vi "ARCO Read Client.vi"() -> ()   [LabVIEW 2017]
uses:
  <vilib>/OPCUA/controls/NodeIds.ctl
  <vilib>/OPCUA/controls/NodeId.ctl
  <vilib>/OPCUA/NI OPC UA Client.lvlib
panel:
  in  "stop":bool
  out "error out":errorcluster
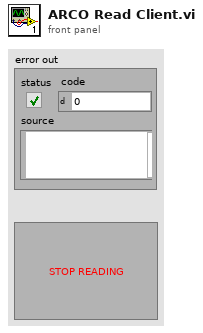
[diagram p1: front panel]
types:
  T1 = cluster{"message mode":enum16{"None", "Sign", "Sign and Encrypt"}, "security":enum16{"Basic256", "Basic128Rsa15"}}
  T2 = typedef "NodeIds.ctl" = T3[]
  T3 = typedef "NodeId.ctl" = string
  T4 = typedef "OPC UA Client Refnum.ctl" = refnum<k21>
  T5 = typedef "Subscription ID.ctl" = u32
  T6 = typedef "Subscription Data Change.ctl" = cluster{"node ID":T3, " value":variant, "timestamp":timestamp, "data type":T7, "status code":T8}
  T7 = typedef "Data Type.ctl" = u16
  T8 = typedef "OPC UA StatusCode.ctl" = u32
  T9 = cluster{"[0]":sgl, "[1]":sgl, "[2]":sgl, "[3]":sgl, "[4]":sgl, "[5]":sgl, "[6]":sgl, "[7]":sgl, "[8]":sgl, "[9]":sgl, "[10]":sgl, "[11]":sgl, "[12]":sgl, "[13]":sgl, "[14]":sgl, "[15]":sgl, "[16]":sgl, "[17]":sgl, "[18]":sgl, "[19]":sgl, "[20]":sgl, "[21]":sgl, "[22]":sgl, "[23]":sgl, "[24]":sgl, "[25]":sgl, "[26]":sgl, "[27]":sgl, "[28]":sgl, "[29]":sgl, "[30]":sgl, "[31]":sgl, "[32]":sgl, "[33]":sgl, "[34]":sgl, "[35]":sgl, "[36]":sgl, "[37]":sgl, "[38]":sgl, "[39]":sgl, "[40]":sgl, "[41]":sgl, "[42]":sgl, "[43]":sgl, "[44]":sgl, "[45]":sgl, "[46]":sgl, "[47]":sgl, "[48]":sgl, "[49]":sgl, "[50]":sgl, "[51]":sgl, "[52]":sgl, "[53]":sgl, "[54]":sgl, "[55]":sgl, "[56]":sgl, "[57]":sgl, "[58]":sgl, "[59]":sgl, "[60]":sgl, "[61]":sgl, "[62]":sgl}
  T10 = cluster{"[0]":bool, "[1]":bool, "[2]":bool, "[3]":bool, "[4]":bool, "[5]":bool, "[6]":bool, "[7]":bool, "[8]":bool, "[9]":bool, "[10]":bool, "[11]":bool, "[12]":bool, "[13]":bool, "[14]":bool, "[15]":bool, "[16]":bool, "[17]":bool, "[18]":bool, "[19]":bool, "[20]":bool, "[21]":bool, "[22]":bool, "[23]":bool, "[24]":bool, "[25]":bool, "[26]":bool, "[27]":bool, "[28]":bool, "[29]":bool, "[30]":bool, "[31]":bool, "[32]":bool, "[33]":bool, "[34]":bool, "[35]":bool, "[36]":bool, "[37]":bool, "[38]":bool, "[39]":bool, "[40]":bool, "[41]":bool, "[42]":bool, "[43]":bool, "[44]":bool, "[45]":bool, "[46]":bool, "[47]":bool, "[48]":bool, "[49]":bool, "[50]":bool, "[51]":bool, "[52]":bool, "[53]":bool, "[54]":bool, "[55]":bool, "[56]":bool, "[57]":bool, "[58]":bool, "[59]":bool, "[60]":bool, "[61]":bool, "[62]":bool}
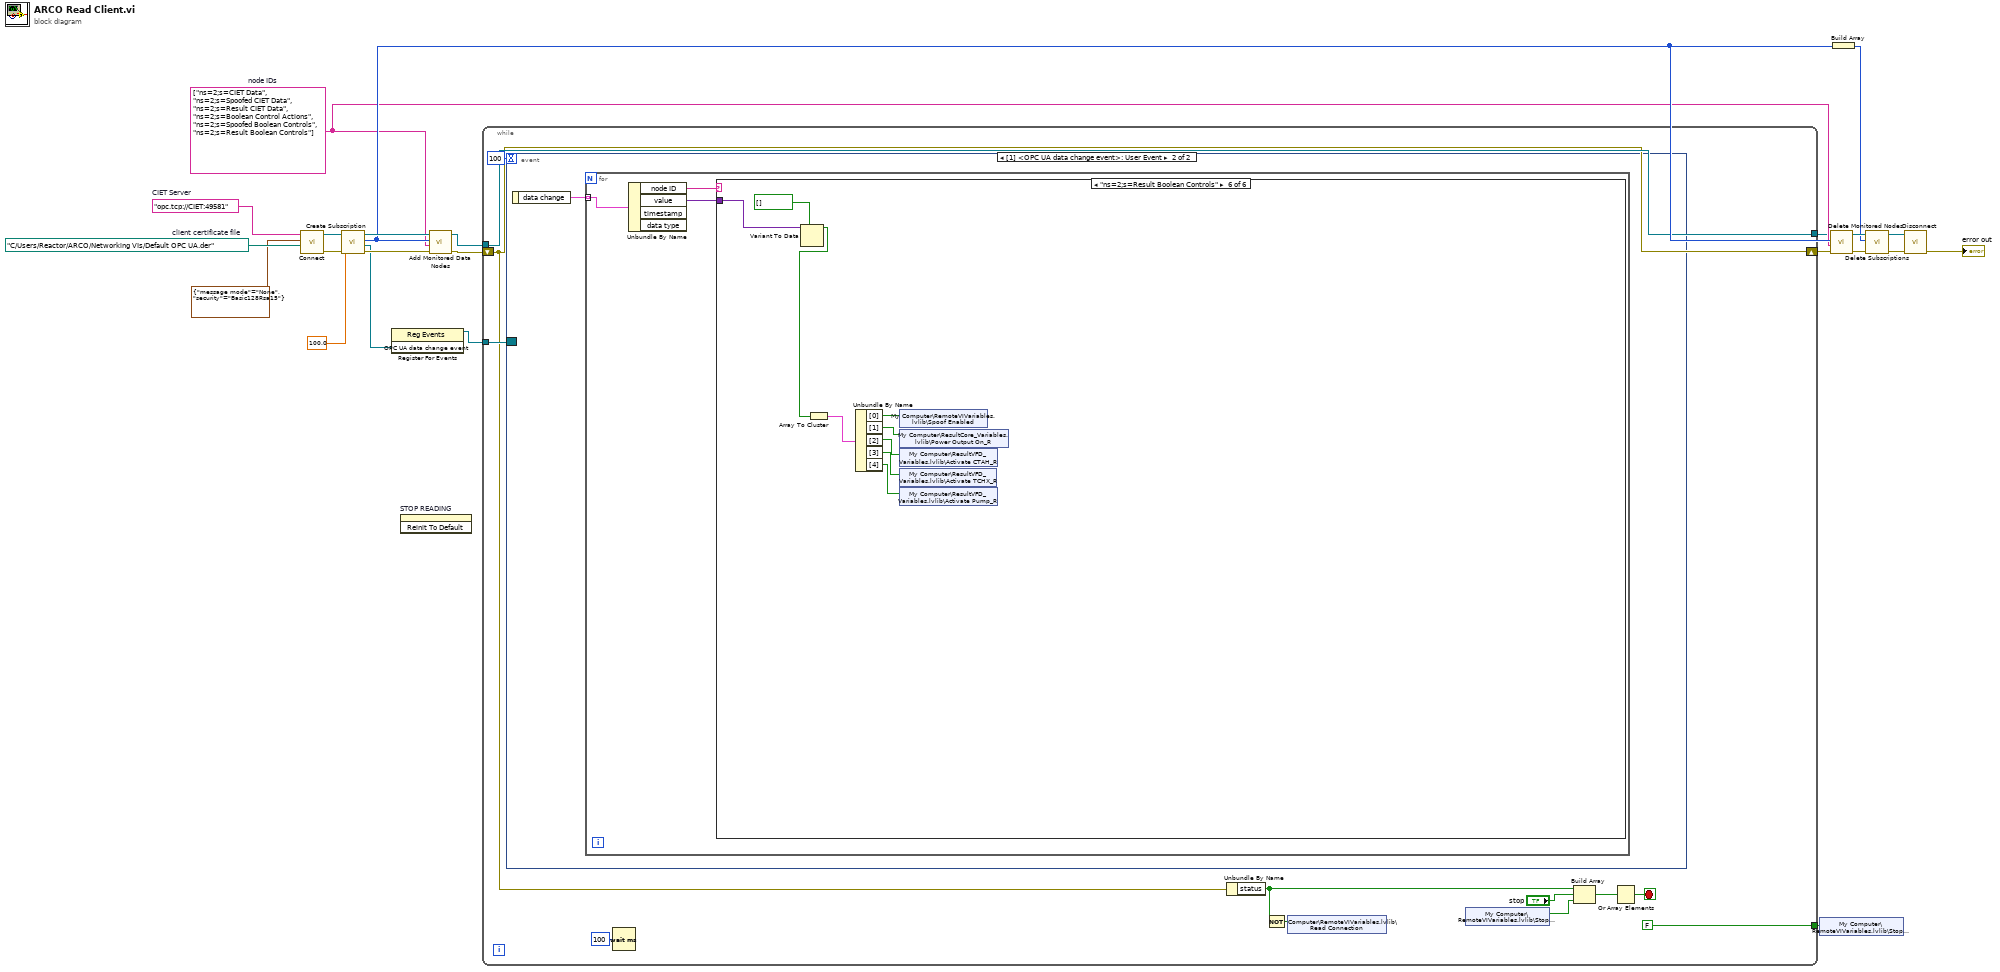
[diagram p0: block diagram]
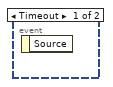
[diagram p2: hidden frame]
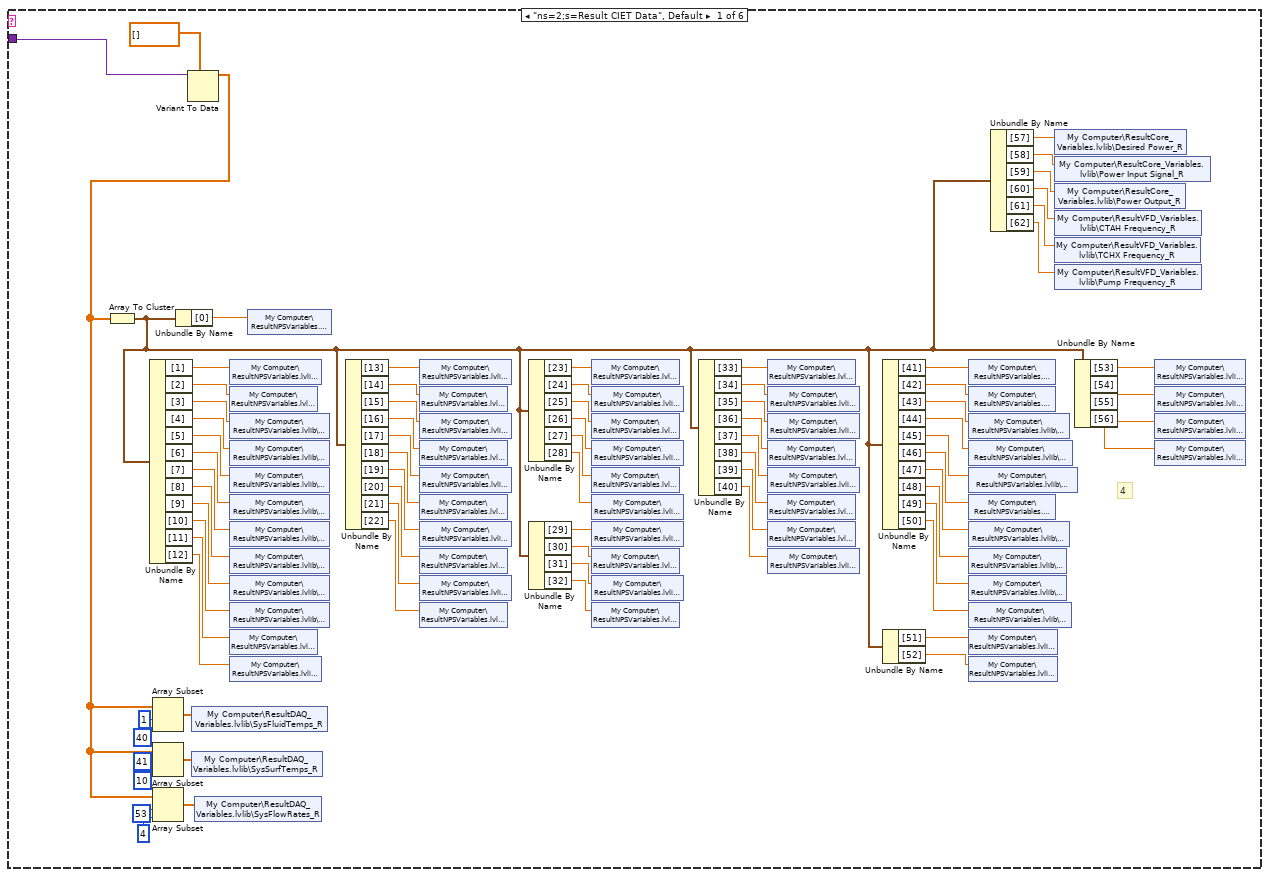
[diagram p3: hidden frame]
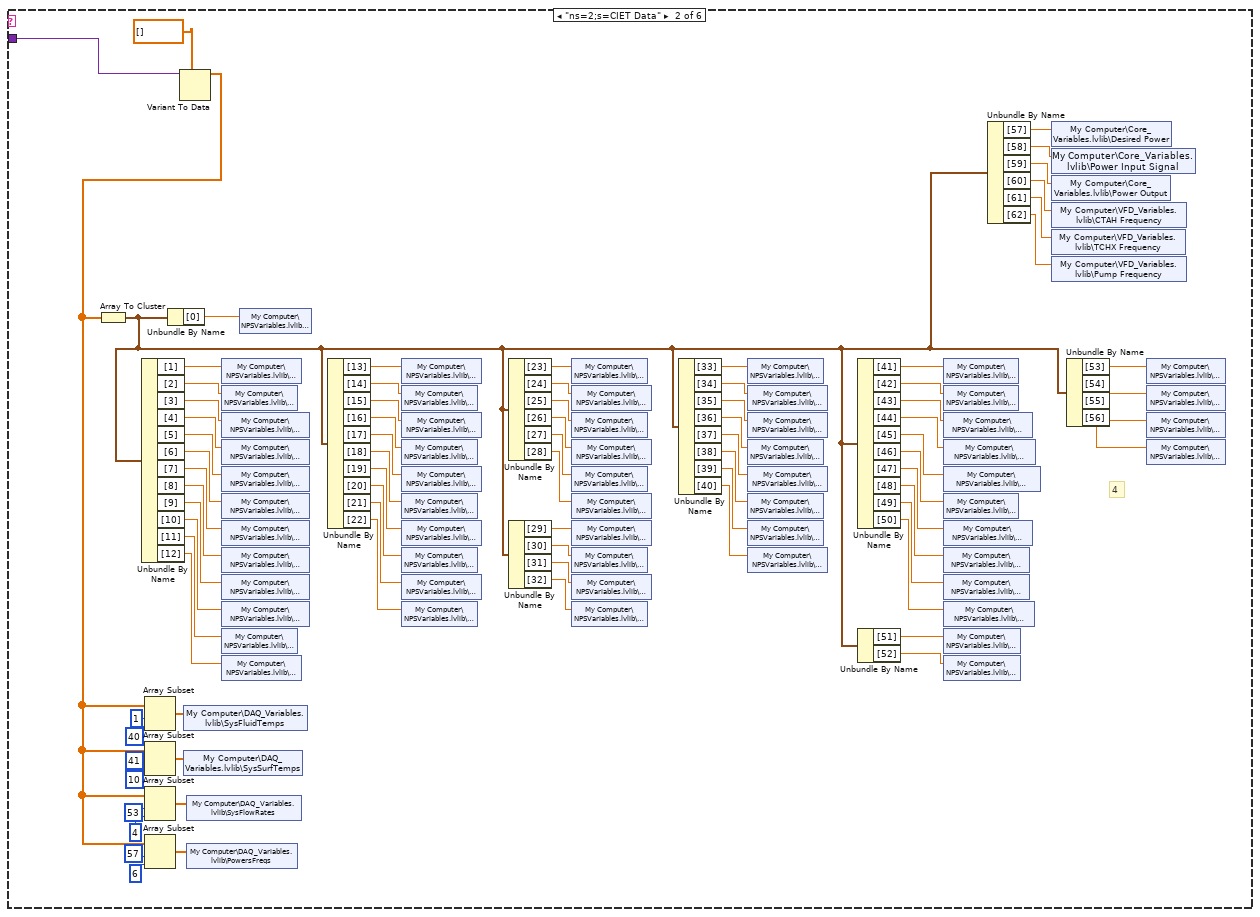
[diagram p4: hidden frame]
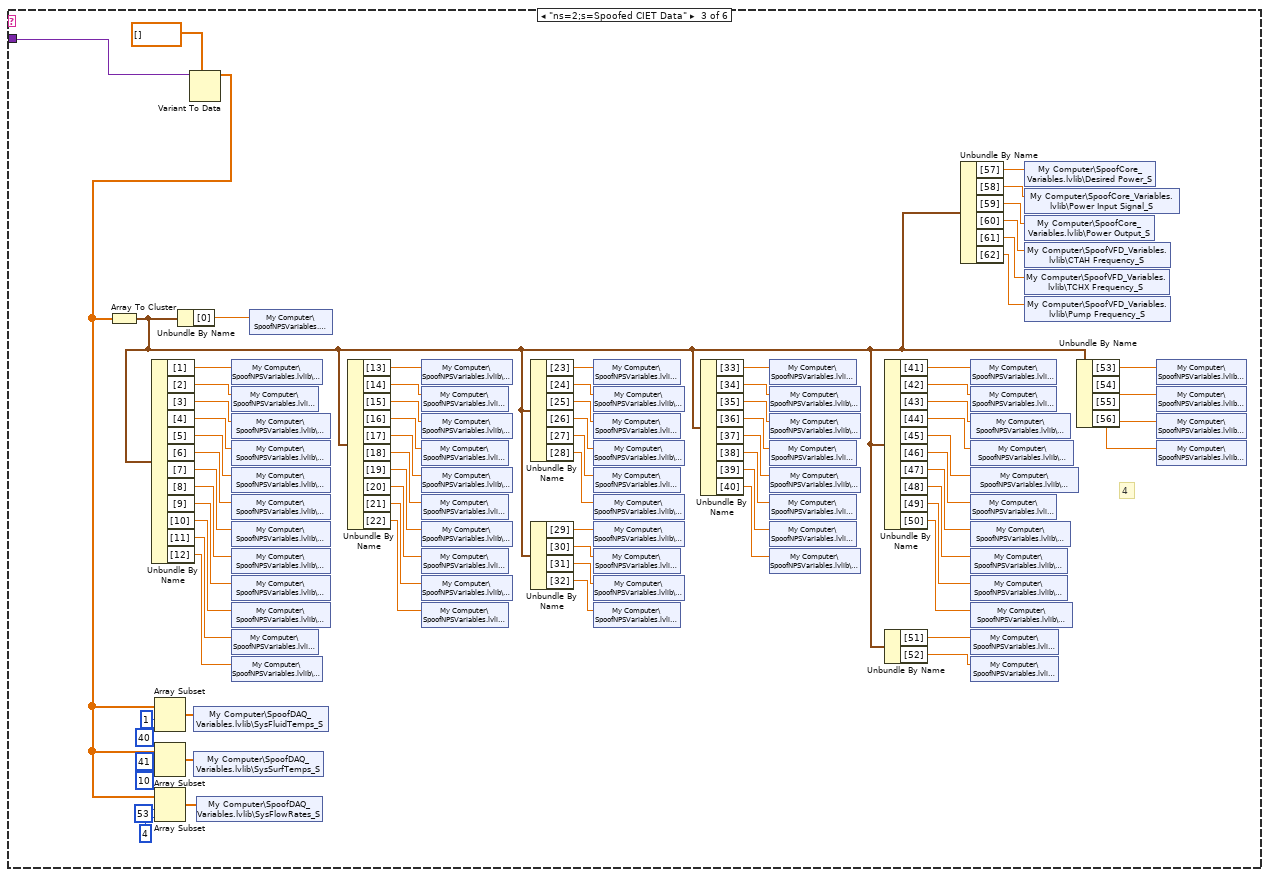
[diagram p5: hidden frame]
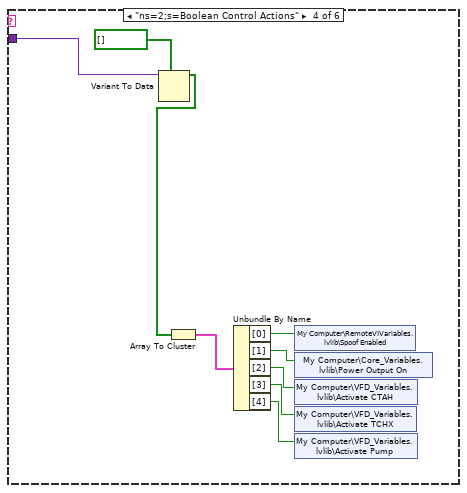
[diagram p6: hidden frame]
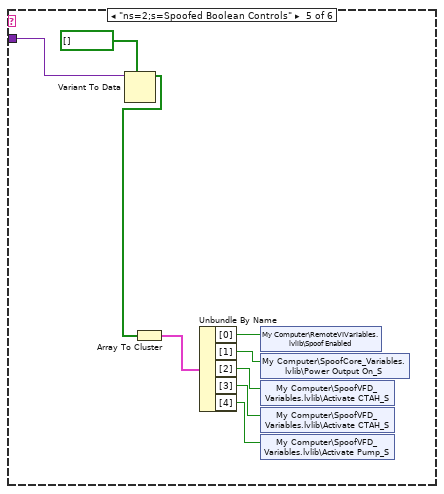
[diagram p7: hidden frame]
diagram:
  w7 = T2 ["ns=2;s=CIET Data", "ns=2;s=Spoofed CIET Data", "ns=2;s=Result CIET Data", "ns=2;s=Boolean Control Actions", "ns=2;s=Spoofed Boolean Controls", "ns=2;s=Result Boolean Controls"]  # node IDs
  w21 = path "C:/Users/Reactor/ARCO/Networking VIs/Default OPC UA.der"  # client certificate file
  w22 = "opc.tcp://CIET:49581"  # CIET Server
  n1 = call <vilib>:"Connect.vi"("client certificate file"=w21, "security policy"=T1 {"message mode"=enum."None", "security"=enum."Basic128Rsa15"}, "server endpoint URL"=w22) -> ("error out"=w3:errorcluster, "OPC UA client refnum out"=w19:T4)  [unwired: 6 in, 1 out]
  n2 = call <vilib>:"Create Subscription.vi"("error in (no error)"=w3, "publishing interval (1000 ms)"=100.0, "OPC UA client refnum in"=w19) -> ("error out"=w17:errorcluster, "OPC UA data change event"=w16:refnum<user-event>, "subscription ID out"=w11:T5, "OPC UA client refnum out"=w18:T4)  [unwired: 4 in, 1 out]
  n3 = register-events(w16) -> (reference out=w9:refnum<event-registration>)  [unwired: 2 in, 1 out]
  n4 = invoke on="STOP READING" class="Bool (strict)" method="Reinit To Default"() -> ()  [unwired: 3 in, 3 out]
  n5 = call <vilib>:"Add Monitored Data Nodes.vi"("error in (no error)"=w17, "node IDs"=w7, "subscription ID in"=w11, "OPC UA client refnum in"=w18) -> ("error out"=w2:errorcluster, "OPC UA client refnum out"=w8:T4)  [unwired: 4 in, 2 out]
  n6 = while {
    tunnel: w9 -> [w35]
    tunnel: w8 -> [w33]
    tunnel: [w33] -> w6
    tunnel: [FALSE] -> w4
    shift-right: [w24] -> w1
    shift-left: w2 -> [w24]
    stop <- w25 stop-if-true
    n7 = event shown="[1] <OPC UA data change event>: User Event" {
      selector: w35 -> [_ _]
      dyn-events: _ -> [_ _]
      timeout: 100 -> [_ _]
      event Timeout {
        n8 = event-data() -> ()  [unwired: 1 in, 1 out]
      }
      event User Event {
        n9 = event-data() -> ("data change"=w36:T6[])  [unwired: 1 in]
        n10 = for {
          tunnel: w36 -> [w38] mode=indexing
          n11 = Unbundle By Name(w38) -> ("node ID"=w37:T3, "value"=w39:variant)  [unwired: 2 out]
          n12 = case shown="\"ns=2;s=Result Boolean Controls\"" w37 {
            tunnel: w39 -> [w49 w135 w203 w271 w280 w289]
            frame "ns=2;s=Result CIET Data", Default {
              # "4"
              n13 = Variant To Data(type=sgl[] [], Variant=w49) -> (data=w47:sgl[])  [unwired: 1 in, 1 out]
              n14 = Array To Cluster(array=w47) -> (cluster=w40:T9)
              n15 = Unbundle By Name(w40) -> ("[1]"=w56:sgl, "[2]"=w58:sgl, "[3]"=w59:sgl, "[4]"=w60:sgl, "[5]"=w61:sgl, "[6]"=w62:sgl, "[7]"=w63:sgl, "[8]"=w64:sgl, "[9]"=w65:sgl, "[10]"=w66:sgl, "[11]"=w67:sgl, "[12]"=w68:sgl)
              n16 = Array Subset(array=w47, index=1, length=40) -> (w113:sgl[])
              n17 = Array Subset(array=w47, index=41, length=10) -> (w114:sgl[])
              n18 = Array Subset(array=w47, index=53, length=4) -> (w115:sgl[])
              n19 = Unbundle By Name(w40) -> ("[0]"=w57:sgl)
              n20 = shared-variable "My Computer\\ResultDAQ_Variables.lvlib\\SysFluidTemps_R"(w113) -> ()  [unwired: 1 in, 1 out]
              n21 = shared-variable "My Computer\\ResultDAQ_Variables.lvlib\\SysSurfTemps_R"(w114) -> ()  [unwired: 1 in, 1 out]
              n22 = shared-variable "My Computer\\ResultDAQ_Variables.lvlib\\SysFlowRates_R"(w115) -> ()  [unwired: 1 in, 1 out]
              n23 = shared-variable "My Computer\\ResultNPSVariables.lvlib\\WT-10_R"(w56) -> ()  [unwired: 1 in, 1 out]
              n24 = shared-variable "My Computer\\ResultNPSVariables.lvlib\\BT-11_R"(w58) -> ()  [unwired: 1 in, 1 out]
              n25 = shared-variable "My Computer\\ResultNPSVariables.lvlib\\CX-10-1_R"(w59) -> ()  [unwired: 1 in, 1 out]
              n26 = shared-variable "My Computer\\ResultNPSVariables.lvlib\\CX-10-2_R"(w60) -> ()  [unwired: 1 in, 1 out]
              n27 = shared-variable "My Computer\\ResultNPSVariables.lvlib\\CX-10-3_R"(w61) -> ()  [unwired: 1 in, 1 out]
              n28 = shared-variable "My Computer\\ResultNPSVariables.lvlib\\CX-10-4_R"(w62) -> ()  [unwired: 1 in, 1 out]
              n29 = shared-variable "My Computer\\ResultNPSVariables.lvlib\\CX-11-1_R"(w63) -> ()  [unwired: 1 in, 1 out]
              n30 = shared-variable "My Computer\\ResultNPSVariables.lvlib\\CX-11-2_R"(w64) -> ()  [unwired: 1 in, 1 out]
              n31 = shared-variable "My Computer\\ResultNPSVariables.lvlib\\CX-11-3_R"(w65) -> ()  [unwired: 1 in, 1 out]
              n32 = shared-variable "My Computer\\ResultNPSVariables.lvlib\\CX-11-4_R"(w66) -> ()  [unwired: 1 in, 1 out]
              n33 = shared-variable "My Computer\\ResultNPSVariables.lvlib\\BT-12_R"(w67) -> ()  [unwired: 1 in, 1 out]
              n34 = shared-variable "My Computer\\ResultNPSVariables.lvlib\\WT-13_R"(w68) -> ()  [unwired: 1 in, 1 out]
              n35 = shared-variable "My Computer\\ResultNPSVariables.lvlib\\Time_R"(w57) -> ()  [unwired: 1 in, 1 out]
              n36 = Unbundle By Name(w40) -> ("[13]"=w69:sgl, "[14]"=w70:sgl, "[15]"=w71:sgl, "[16]"=w72:sgl, "[17]"=w73:sgl, "[18]"=w74:sgl, "[19]"=w75:sgl, "[20]"=w76:sgl, "[21]"=w77:sgl, "[22]"=w78:sgl)
              n37 = shared-variable "My Computer\\ResultNPSVariables.lvlib\\WT-20_R"(w69) -> ()  [unwired: 1 in, 1 out]
              n38 = shared-variable "My Computer\\ResultNPSVariables.lvlib\\BT-21_R"(w70) -> ()  [unwired: 1 in, 1 out]
              n39 = shared-variable "My Computer\\ResultNPSVariables.lvlib\\WT-22_R"(w71) -> ()  [unwired: 1 in, 1 out]
              n40 = shared-variable "My Computer\\ResultNPSVariables.lvlib\\BT-23_R"(w72) -> ()  [unwired: 1 in, 1 out]
              n41 = shared-variable "My Computer\\ResultNPSVariables.lvlib\\WT-24_R"(w73) -> ()  [unwired: 1 in, 1 out]
              n42 = shared-variable "My Computer\\ResultNPSVariables.lvlib\\BT-25_R"(w74) -> ()  [unwired: 1 in, 1 out]
              n43 = shared-variable "My Computer\\ResultNPSVariables.lvlib\\WT-26_R"(w75) -> ()  [unwired: 1 in, 1 out]
              n44 = shared-variable "My Computer\\ResultNPSVariables.lvlib\\BT-27_R"(w76) -> ()  [unwired: 1 in, 1 out]
              n45 = shared-variable "My Computer\\ResultNPSVariables.lvlib\\WT-28_R"(w77) -> ()  [unwired: 1 in, 1 out]
              n46 = shared-variable "My Computer\\ResultNPSVariables.lvlib\\BT-29_R"(w78) -> ()  [unwired: 1 in, 1 out]
              n47 = Unbundle By Name(w40) -> ("[23]"=w79:sgl, "[24]"=w80:sgl, "[25]"=w81:sgl, "[26]"=w82:sgl, "[27]"=w83:sgl, "[28]"=w84:sgl)
              n48 = Unbundle By Name(w40) -> ("[29]"=w85:sgl, "[30]"=w86:sgl, "[31]"=w87:sgl, "[32]"=w88:sgl)
              n49 = shared-variable "My Computer\\ResultNPSVariables.lvlib\\BT-30_R"(w79) -> ()  [unwired: 1 in, 1 out]
              n50 = shared-variable "My Computer\\ResultNPSVariables.lvlib\\WT-31_R"(w80) -> ()  [unwired: 1 in, 1 out]
              n51 = shared-variable "My Computer\\ResultNPSVariables.lvlib\\BT-32_R"(w81) -> ()  [unwired: 1 in, 1 out]
              n52 = shared-variable "My Computer\\ResultNPSVariables.lvlib\\WT-33_R"(w82) -> ()  [unwired: 1 in, 1 out]
              n53 = shared-variable "My Computer\\ResultNPSVariables.lvlib\\BT-34_R"(w83) -> ()  [unwired: 1 in, 1 out]
              n54 = shared-variable "My Computer\\ResultNPSVariables.lvlib\\WT-35_R"(w84) -> ()  [unwired: 1 in, 1 out]
              n55 = shared-variable "My Computer\\ResultNPSVariables.lvlib\\WT-40_R"(w85) -> ()  [unwired: 1 in, 1 out]
              n56 = shared-variable "My Computer\\ResultNPSVariables.lvlib\\BT-41_R"(w86) -> ()  [unwired: 1 in, 1 out]
              n57 = shared-variable "My Computer\\ResultNPSVariables.lvlib\\WT-42_R"(w87) -> ()  [unwired: 1 in, 1 out]
              n58 = shared-variable "My Computer\\ResultNPSVariables.lvlib\\BT-43_R"(w88) -> ()  [unwired: 1 in, 1 out]
              n59 = Unbundle By Name(w40) -> ("[33]"=w89:sgl, "[34]"=w90:sgl, "[35]"=w91:sgl, "[36]"=w92:sgl, "[37]"=w93:sgl, "[38]"=w94:sgl, "[39]"=w95:sgl, "[40]"=w96:sgl)
              n60 = shared-variable "My Computer\\ResultNPSVariables.lvlib\\BT-60_R"(w89) -> ()  [unwired: 1 in, 1 out]
              n61 = shared-variable "My Computer\\ResultNPSVariables.lvlib\\WT-61_R"(w90) -> ()  [unwired: 1 in, 1 out]
              n62 = shared-variable "My Computer\\ResultNPSVariables.lvlib\\WT-62_R"(w91) -> ()  [unwired: 1 in, 1 out]
              n63 = shared-variable "My Computer\\ResultNPSVariables.lvlib\\BT-63_R"(w92) -> ()  [unwired: 1 in, 1 out]
              n64 = shared-variable "My Computer\\ResultNPSVariables.lvlib\\WT-64_R"(w93) -> ()  [unwired: 1 in, 1 out]
              n65 = shared-variable "My Computer\\ResultNPSVariables.lvlib\\BT-65_R"(w94) -> ()  [unwired: 1 in, 1 out]
              n66 = shared-variable "My Computer\\ResultNPSVariables.lvlib\\BT-66_R"(w95) -> ()  [unwired: 1 in, 1 out]
              n67 = shared-variable "My Computer\\ResultNPSVariables.lvlib\\WT-67_R"(w96) -> ()  [unwired: 1 in, 1 out]
              n68 = Unbundle By Name(w40) -> ("[41]"=w97:sgl, "[42]"=w98:sgl, "[43]"=w99:sgl, "[44]"=w100:sgl, "[45]"=w101:sgl, "[46]"=w102:sgl, "[47]"=w103:sgl, "[48]"=w104:sgl, "[49]"=w105:sgl, "[50]"=w106:sgl)
              n69 = Unbundle By Name(w40) -> ("[51]"=w107:sgl, "[52]"=w108:sgl)
              n70 = shared-variable "My Computer\\ResultNPSVariables.lvlib\\ST-10_R"(w97) -> ()  [unwired: 1 in, 1 out]
              n71 = shared-variable "My Computer\\ResultNPSVariables.lvlib\\ST-11_R"(w98) -> ()  [unwired: 1 in, 1 out]
              n72 = shared-variable "My Computer\\ResultNPSVariables.lvlib\\ST-12-N_R"(w99) -> ()  [unwired: 1 in, 1 out]
              n73 = shared-variable "My Computer\\ResultNPSVariables.lvlib\\ST-12-SE_R"(w100) -> ()  [unwired: 1 in, 1 out]
              n74 = shared-variable "My Computer\\ResultNPSVariables.lvlib\\ST-12-SW_R"(w101) -> ()  [unwired: 1 in, 1 out]
              n75 = shared-variable "My Computer\\ResultNPSVariables.lvlib\\ST-13_R"(w102) -> ()  [unwired: 1 in, 1 out]
              n76 = shared-variable "My Computer\\ResultNPSVariables.lvlib\\ST-14-N_R"(w103) -> ()  [unwired: 1 in, 1 out]
              n77 = shared-variable "My Computer\\ResultNPSVariables.lvlib\\ST-14-E_R"(w104) -> ()  [unwired: 1 in, 1 out]
              n78 = shared-variable "My Computer\\ResultNPSVariables.lvlib\\ST-14-S_R"(w105) -> ()  [unwired: 1 in, 1 out]
              n79 = shared-variable "My Computer\\ResultNPSVariables.lvlib\\ST-14-W_R"(w106) -> ()  [unwired: 1 in, 1 out]
              n80 = shared-variable "My Computer\\ResultNPSVariables.lvlib\\AT-01_R"(w107) -> ()  [unwired: 1 in, 1 out]
              n81 = shared-variable "My Computer\\ResultNPSVariables.lvlib\\AT-02_R"(w108) -> ()  [unwired: 1 in, 1 out]
              n82 = Unbundle By Name(w40) -> ("[57]"=w46:sgl, "[58]"=w45:sgl, "[59]"=w44:sgl, "[60]"=w43:sgl, "[61]"=w42:sgl, "[62]"=w41:sgl)
              n83 = shared-variable "My Computer\\ResultCore_Variables.lvlib\\Desired Power_R"(w46) -> ()  [unwired: 1 in, 1 out]
              n84 = shared-variable "My Computer\\ResultCore_Variables.lvlib\\Power Input Signal_R"(w45) -> ()  [unwired: 1 in, 1 out]
              n85 = shared-variable "My Computer\\ResultCore_Variables.lvlib\\Power Output_R"(w44) -> ()  [unwired: 1 in, 1 out]
              n86 = shared-variable "My Computer\\ResultVFD_Variables.lvlib\\CTAH Frequency_R"(w43) -> ()  [unwired: 1 in, 1 out]
              n87 = shared-variable "My Computer\\ResultVFD_Variables.lvlib\\TCHX Frequency_R"(w42) -> ()  [unwired: 1 in, 1 out]
              n88 = shared-variable "My Computer\\ResultVFD_Variables.lvlib\\Pump Frequency_R"(w41) -> ()  [unwired: 1 in, 1 out]
              n89 = Unbundle By Name(w40) -> ("[53]"=w109:sgl, "[54]"=w110:sgl, "[55]"=w111:sgl, "[56]"=w112:sgl)
              n90 = shared-variable "My Computer\\ResultNPSVariables.lvlib\\FM-20_R"(w109) -> ()  [unwired: 1 in, 1 out]
              n91 = shared-variable "My Computer\\ResultNPSVariables.lvlib\\FM-30_R"(w110) -> ()  [unwired: 1 in, 1 out]
              n92 = shared-variable "My Computer\\ResultNPSVariables.lvlib\\FM-40_R"(w111) -> ()  [unwired: 1 in, 1 out]
              n93 = shared-variable "My Computer\\ResultNPSVariables.lvlib\\FM-60_R"(w112) -> ()  [unwired: 1 in, 1 out]
            }
            frame "ns=2;s=CIET Data" {
              # "4"
              n94 = Variant To Data(type=sgl[] [], Variant=w135) -> (data=w117:sgl[])  [unwired: 1 in, 1 out]
              n95 = Array To Cluster(array=w117) -> (cluster=w116:T9)
              n96 = Unbundle By Name(w116) -> ("[1]"=w134:sgl, "[2]"=w137:sgl, "[3]"=w138:sgl, "[4]"=w139:sgl, "[5]"=w140:sgl, "[6]"=w141:sgl, "[7]"=w142:sgl, "[8]"=w143:sgl, "[9]"=w144:sgl, "[10]"=w145:sgl, "[11]"=w146:sgl, "[12]"=w147:sgl)
              n97 = Array Subset(array=w117, index=1, length=40) -> (w192:sgl[])
              n98 = Array Subset(array=w117, index=41, length=10) -> (w193:sgl[])
              n99 = Array Subset(array=w117, index=53, length=4) -> (w194:sgl[])
              n100 = Array Subset(array=w117, index=57, length=6) -> (w124:sgl[])
              n101 = Unbundle By Name(w116) -> ("[0]"=w136:sgl)
              n102 = shared-variable "My Computer\\DAQ_Variables.lvlib\\SysFluidTemps"(w192) -> ()  [unwired: 1 in, 1 out]
              n103 = shared-variable "My Computer\\DAQ_Variables.lvlib\\SysSurfTemps"(w193) -> ()  [unwired: 1 in, 1 out]
              n104 = shared-variable "My Computer\\DAQ_Variables.lvlib\\SysFlowRates"(w194) -> ()  [unwired: 1 in, 1 out]
              n105 = shared-variable "My Computer\\DAQ_Variables.lvlib\\PowersFreqs"(w124) -> ()  [unwired: 1 in, 1 out]
              n106 = shared-variable "My Computer\\NPSVariables.lvlib\\WT-10"(w134) -> ()  [unwired: 1 in, 1 out]
              n107 = shared-variable "My Computer\\NPSVariables.lvlib\\BT-11"(w137) -> ()  [unwired: 1 in, 1 out]
              n108 = shared-variable "My Computer\\NPSVariables.lvlib\\CX-10-1"(w138) -> ()  [unwired: 1 in, 1 out]
              n109 = shared-variable "My Computer\\NPSVariables.lvlib\\CX-10-2"(w139) -> ()  [unwired: 1 in, 1 out]
              n110 = shared-variable "My Computer\\NPSVariables.lvlib\\CX-10-3"(w140) -> ()  [unwired: 1 in, 1 out]
              n111 = shared-variable "My Computer\\NPSVariables.lvlib\\CX-10-4"(w141) -> ()  [unwired: 1 in, 1 out]
              n112 = shared-variable "My Computer\\NPSVariables.lvlib\\CX-11-1"(w142) -> ()  [unwired: 1 in, 1 out]
              n113 = shared-variable "My Computer\\NPSVariables.lvlib\\CX-11-2"(w143) -> ()  [unwired: 1 in, 1 out]
              n114 = shared-variable "My Computer\\NPSVariables.lvlib\\CX-11-3"(w144) -> ()  [unwired: 1 in, 1 out]
              n115 = shared-variable "My Computer\\NPSVariables.lvlib\\CX-11-4"(w145) -> ()  [unwired: 1 in, 1 out]
              n116 = shared-variable "My Computer\\NPSVariables.lvlib\\BT-12"(w146) -> ()  [unwired: 1 in, 1 out]
              n117 = shared-variable "My Computer\\NPSVariables.lvlib\\WT-13"(w147) -> ()  [unwired: 1 in, 1 out]
              n118 = shared-variable "My Computer\\NPSVariables.lvlib\\Time"(w136) -> ()  [unwired: 1 in, 1 out]
              n119 = Unbundle By Name(w116) -> ("[13]"=w148:sgl, "[14]"=w149:sgl, "[15]"=w150:sgl, "[16]"=w151:sgl, "[17]"=w152:sgl, "[18]"=w153:sgl, "[19]"=w154:sgl, "[20]"=w155:sgl, "[21]"=w156:sgl, "[22]"=w157:sgl)
              n120 = shared-variable "My Computer\\NPSVariables.lvlib\\WT-20"(w148) -> ()  [unwired: 1 in, 1 out]
              n121 = shared-variable "My Computer\\NPSVariables.lvlib\\BT-21"(w149) -> ()  [unwired: 1 in, 1 out]
              n122 = shared-variable "My Computer\\NPSVariables.lvlib\\WT-22"(w150) -> ()  [unwired: 1 in, 1 out]
              n123 = shared-variable "My Computer\\NPSVariables.lvlib\\BT-23"(w151) -> ()  [unwired: 1 in, 1 out]
              n124 = shared-variable "My Computer\\NPSVariables.lvlib\\WT-24"(w152) -> ()  [unwired: 1 in, 1 out]
              n125 = shared-variable "My Computer\\NPSVariables.lvlib\\BT-25"(w153) -> ()  [unwired: 1 in, 1 out]
              n126 = shared-variable "My Computer\\NPSVariables.lvlib\\WT-26"(w154) -> ()  [unwired: 1 in, 1 out]
              n127 = shared-variable "My Computer\\NPSVariables.lvlib\\BT-27"(w155) -> ()  [unwired: 1 in, 1 out]
              n128 = shared-variable "My Computer\\NPSVariables.lvlib\\WT-28"(w156) -> ()  [unwired: 1 in, 1 out]
              n129 = shared-variable "My Computer\\NPSVariables.lvlib\\BT-29"(w157) -> ()  [unwired: 1 in, 1 out]
              n130 = Unbundle By Name(w116) -> ("[23]"=w158:sgl, "[24]"=w159:sgl, "[25]"=w160:sgl, "[26]"=w161:sgl, "[27]"=w162:sgl, "[28]"=w163:sgl)
              n131 = Unbundle By Name(w116) -> ("[29]"=w164:sgl, "[30]"=w165:sgl, "[31]"=w166:sgl, "[32]"=w167:sgl)
              n132 = shared-variable "My Computer\\NPSVariables.lvlib\\BT-30"(w158) -> ()  [unwired: 1 in, 1 out]
              n133 = shared-variable "My Computer\\NPSVariables.lvlib\\WT-31"(w159) -> ()  [unwired: 1 in, 1 out]
              n134 = shared-variable "My Computer\\NPSVariables.lvlib\\BT-32"(w160) -> ()  [unwired: 1 in, 1 out]
              n135 = shared-variable "My Computer\\NPSVariables.lvlib\\WT-33"(w161) -> ()  [unwired: 1 in, 1 out]
              n136 = shared-variable "My Computer\\NPSVariables.lvlib\\BT-34"(w162) -> ()  [unwired: 1 in, 1 out]
              n137 = shared-variable "My Computer\\NPSVariables.lvlib\\WT-35"(w163) -> ()  [unwired: 1 in, 1 out]
              n138 = shared-variable "My Computer\\NPSVariables.lvlib\\WT-40"(w164) -> ()  [unwired: 1 in, 1 out]
              n139 = shared-variable "My Computer\\NPSVariables.lvlib\\BT-41"(w165) -> ()  [unwired: 1 in, 1 out]
              n140 = shared-variable "My Computer\\NPSVariables.lvlib\\WT-42"(w166) -> ()  [unwired: 1 in, 1 out]
              n141 = shared-variable "My Computer\\NPSVariables.lvlib\\BT-43"(w167) -> ()  [unwired: 1 in, 1 out]
              n142 = Unbundle By Name(w116) -> ("[33]"=w168:sgl, "[34]"=w169:sgl, "[35]"=w170:sgl, "[36]"=w171:sgl, "[37]"=w172:sgl, "[38]"=w173:sgl, "[39]"=w174:sgl, "[40]"=w175:sgl)
              n143 = shared-variable "My Computer\\NPSVariables.lvlib\\BT-60"(w168) -> ()  [unwired: 1 in, 1 out]
              n144 = shared-variable "My Computer\\NPSVariables.lvlib\\WT-61"(w169) -> ()  [unwired: 1 in, 1 out]
              n145 = shared-variable "My Computer\\NPSVariables.lvlib\\WT-62"(w170) -> ()  [unwired: 1 in, 1 out]
              n146 = shared-variable "My Computer\\NPSVariables.lvlib\\BT-63"(w171) -> ()  [unwired: 1 in, 1 out]
              n147 = shared-variable "My Computer\\NPSVariables.lvlib\\WT-64"(w172) -> ()  [unwired: 1 in, 1 out]
              n148 = shared-variable "My Computer\\NPSVariables.lvlib\\BT-65"(w173) -> ()  [unwired: 1 in, 1 out]
              n149 = shared-variable "My Computer\\NPSVariables.lvlib\\BT-66"(w174) -> ()  [unwired: 1 in, 1 out]
              n150 = shared-variable "My Computer\\NPSVariables.lvlib\\WT-67"(w175) -> ()  [unwired: 1 in, 1 out]
              n151 = Unbundle By Name(w116) -> ("[41]"=w176:sgl, "[42]"=w177:sgl, "[43]"=w178:sgl, "[44]"=w179:sgl, "[45]"=w180:sgl, "[46]"=w181:sgl, "[47]"=w182:sgl, "[48]"=w183:sgl, "[49]"=w184:sgl, "[50]"=w185:sgl)
              n152 = Unbundle By Name(w116) -> ("[51]"=w186:sgl, "[52]"=w187:sgl)
              n153 = shared-variable "My Computer\\NPSVariables.lvlib\\ST-10"(w176) -> ()  [unwired: 1 in, 1 out]
              n154 = shared-variable "My Computer\\NPSVariables.lvlib\\ST-11"(w177) -> ()  [unwired: 1 in, 1 out]
              n155 = shared-variable "My Computer\\NPSVariables.lvlib\\ST-12-N"(w178) -> ()  [unwired: 1 in, 1 out]
              n156 = shared-variable "My Computer\\NPSVariables.lvlib\\ST-12-SE"(w179) -> ()  [unwired: 1 in, 1 out]
              n157 = shared-variable "My Computer\\NPSVariables.lvlib\\ST-12-SW"(w180) -> ()  [unwired: 1 in, 1 out]
              n158 = shared-variable "My Computer\\NPSVariables.lvlib\\ST-13"(w181) -> ()  [unwired: 1 in, 1 out]
              n159 = shared-variable "My Computer\\NPSVariables.lvlib\\ST-14-N"(w182) -> ()  [unwired: 1 in, 1 out]
              n160 = shared-variable "My Computer\\NPSVariables.lvlib\\ST-14-E"(w183) -> ()  [unwired: 1 in, 1 out]
              n161 = shared-variable "My Computer\\NPSVariables.lvlib\\ST-14-S"(w184) -> ()  [unwired: 1 in, 1 out]
              n162 = shared-variable "My Computer\\NPSVariables.lvlib\\ST-14-W"(w185) -> ()  [unwired: 1 in, 1 out]
              n163 = shared-variable "My Computer\\NPSVariables.lvlib\\AT-01"(w186) -> ()  [unwired: 1 in, 1 out]
              n164 = shared-variable "My Computer\\NPSVariables.lvlib\\AT-02"(w187) -> ()  [unwired: 1 in, 1 out]
              n165 = Unbundle By Name(w116) -> ("[57]"=w123:sgl, "[58]"=w122:sgl, "[59]"=w121:sgl, "[60]"=w120:sgl, "[61]"=w119:sgl, "[62]"=w118:sgl)
              n166 = shared-variable "My Computer\\Core_Variables.lvlib\\Desired Power"(w123) -> ()  [unwired: 1 in, 1 out]
              n167 = shared-variable "My Computer\\Core_Variables.lvlib\\Power Input Signal"(w122) -> ()  [unwired: 1 in, 1 out]
              n168 = shared-variable "My Computer\\Core_Variables.lvlib\\Power Output"(w121) -> ()  [unwired: 1 in, 1 out]
              n169 = shared-variable "My Computer\\VFD_Variables.lvlib\\CTAH Frequency"(w120) -> ()  [unwired: 1 in, 1 out]
              n170 = shared-variable "My Computer\\VFD_Variables.lvlib\\TCHX Frequency"(w119) -> ()  [unwired: 1 in, 1 out]
              n171 = shared-variable "My Computer\\VFD_Variables.lvlib\\Pump Frequency"(w118) -> ()  [unwired: 1 in, 1 out]
              n172 = Unbundle By Name(w116) -> ("[53]"=w188:sgl, "[54]"=w189:sgl, "[55]"=w190:sgl, "[56]"=w191:sgl)
              n173 = shared-variable "My Computer\\NPSVariables.lvlib\\FM-20"(w188) -> ()  [unwired: 1 in, 1 out]
              n174 = shared-variable "My Computer\\NPSVariables.lvlib\\FM-30"(w189) -> ()  [unwired: 1 in, 1 out]
              n175 = shared-variable "My Computer\\NPSVariables.lvlib\\FM-40"(w190) -> ()  [unwired: 1 in, 1 out]
              n176 = shared-variable "My Computer\\NPSVariables.lvlib\\FM-60"(w191) -> ()  [unwired: 1 in, 1 out]
            }
            frame "ns=2;s=Spoofed CIET Data" {
              # "4"
              n177 = Variant To Data(type=sgl[] [], Variant=w203) -> (data=w202:sgl[])  [unwired: 1 in, 1 out]
              n178 = Array To Cluster(array=w202) -> (cluster=w195:T9)
              n179 = Unbundle By Name(w195) -> ("[1]"=w211:sgl, "[2]"=w213:sgl, "[3]"=w214:sgl, "[4]"=w215:sgl, "[5]"=w216:sgl, "[6]"=w217:sgl, "[7]"=w218:sgl, "[8]"=w219:sgl, "[9]"=w220:sgl, "[10]"=w221:sgl, "[11]"=w222:sgl, "[12]"=w223:sgl)
              n180 = Array Subset(array=w202, index=1, length=40) -> (w268:sgl[])
              n181 = Array Subset(array=w202, index=41, length=10) -> (w269:sgl[])
              n182 = Array Subset(array=w202, index=53, length=4) -> (w270:sgl[])
              n183 = Unbundle By Name(w195) -> ("[0]"=w212:sgl)
              n184 = shared-variable "My Computer\\SpoofDAQ_Variables.lvlib\\SysFluidTemps_S"(w268) -> ()  [unwired: 1 in, 1 out]
              n185 = shared-variable "My Computer\\SpoofDAQ_Variables.lvlib\\SysSurfTemps_S"(w269) -> ()  [unwired: 1 in, 1 out]
              n186 = shared-variable "My Computer\\SpoofDAQ_Variables.lvlib\\SysFlowRates_S"(w270) -> ()  [unwired: 1 in, 1 out]
              n187 = shared-variable "My Computer\\SpoofNPSVariables.lvlib\\WT-10_S"(w211) -> ()  [unwired: 1 in, 1 out]
              n188 = shared-variable "My Computer\\SpoofNPSVariables.lvlib\\BT-11_S"(w213) -> ()  [unwired: 1 in, 1 out]
              n189 = shared-variable "My Computer\\SpoofNPSVariables.lvlib\\CX-10-1_S"(w214) -> ()  [unwired: 1 in, 1 out]
              n190 = shared-variable "My Computer\\SpoofNPSVariables.lvlib\\CX-10-2_S"(w215) -> ()  [unwired: 1 in, 1 out]
              n191 = shared-variable "My Computer\\SpoofNPSVariables.lvlib\\CX-10-3_S"(w216) -> ()  [unwired: 1 in, 1 out]
              n192 = shared-variable "My Computer\\SpoofNPSVariables.lvlib\\CX-10-4_S"(w217) -> ()  [unwired: 1 in, 1 out]
              n193 = shared-variable "My Computer\\SpoofNPSVariables.lvlib\\CX-11-1_S"(w218) -> ()  [unwired: 1 in, 1 out]
              n194 = shared-variable "My Computer\\SpoofNPSVariables.lvlib\\CX-11-2_S"(w219) -> ()  [unwired: 1 in, 1 out]
              n195 = shared-variable "My Computer\\SpoofNPSVariables.lvlib\\CX-11-3_S"(w220) -> ()  [unwired: 1 in, 1 out]
              n196 = shared-variable "My Computer\\SpoofNPSVariables.lvlib\\CX-11-4_S"(w221) -> ()  [unwired: 1 in, 1 out]
              n197 = shared-variable "My Computer\\SpoofNPSVariables.lvlib\\BT-12_S"(w222) -> ()  [unwired: 1 in, 1 out]
              n198 = shared-variable "My Computer\\SpoofNPSVariables.lvlib\\WT-13_S"(w223) -> ()  [unwired: 1 in, 1 out]
              n199 = shared-variable "My Computer\\SpoofNPSVariables.lvlib\\Time_S"(w212) -> ()  [unwired: 1 in, 1 out]
              n200 = Unbundle By Name(w195) -> ("[13]"=w224:sgl, "[14]"=w225:sgl, "[15]"=w226:sgl, "[16]"=w227:sgl, "[17]"=w228:sgl, "[18]"=w229:sgl, "[19]"=w230:sgl, "[20]"=w231:sgl, "[21]"=w232:sgl, "[22]"=w233:sgl)
              n201 = shared-variable "My Computer\\SpoofNPSVariables.lvlib\\WT-20_S"(w224) -> ()  [unwired: 1 in, 1 out]
              n202 = shared-variable "My Computer\\SpoofNPSVariables.lvlib\\BT-21_S"(w225) -> ()  [unwired: 1 in, 1 out]
              n203 = shared-variable "My Computer\\SpoofNPSVariables.lvlib\\WT-22_S"(w226) -> ()  [unwired: 1 in, 1 out]
              n204 = shared-variable "My Computer\\SpoofNPSVariables.lvlib\\BT-23_S"(w227) -> ()  [unwired: 1 in, 1 out]
              n205 = shared-variable "My Computer\\SpoofNPSVariables.lvlib\\WT-24_S"(w228) -> ()  [unwired: 1 in, 1 out]
              n206 = shared-variable "My Computer\\SpoofNPSVariables.lvlib\\BT-25_S"(w229) -> ()  [unwired: 1 in, 1 out]
              n207 = shared-variable "My Computer\\SpoofNPSVariables.lvlib\\WT-26_S"(w230) -> ()  [unwired: 1 in, 1 out]
              n208 = shared-variable "My Computer\\SpoofNPSVariables.lvlib\\BT-27_S"(w231) -> ()  [unwired: 1 in, 1 out]
              n209 = shared-variable "My Computer\\SpoofNPSVariables.lvlib\\WT-28_S"(w232) -> ()  [unwired: 1 in, 1 out]
              n210 = shared-variable "My Computer\\SpoofNPSVariables.lvlib\\BT-29_S"(w233) -> ()  [unwired: 1 in, 1 out]
              n211 = Unbundle By Name(w195) -> ("[23]"=w234:sgl, "[24]"=w235:sgl, "[25]"=w236:sgl, "[26]"=w237:sgl, "[27]"=w238:sgl, "[28]"=w239:sgl)
              n212 = Unbundle By Name(w195) -> ("[29]"=w240:sgl, "[30]"=w241:sgl, "[31]"=w242:sgl, "[32]"=w243:sgl)
              n213 = shared-variable "My Computer\\SpoofNPSVariables.lvlib\\BT-30_S"(w234) -> ()  [unwired: 1 in, 1 out]
              n214 = shared-variable "My Computer\\SpoofNPSVariables.lvlib\\WT-31_S"(w235) -> ()  [unwired: 1 in, 1 out]
              n215 = shared-variable "My Computer\\SpoofNPSVariables.lvlib\\BT-32_S"(w236) -> ()  [unwired: 1 in, 1 out]
              n216 = shared-variable "My Computer\\SpoofNPSVariables.lvlib\\WT-33_S"(w237) -> ()  [unwired: 1 in, 1 out]
              n217 = shared-variable "My Computer\\SpoofNPSVariables.lvlib\\BT-34_S"(w238) -> ()  [unwired: 1 in, 1 out]
              n218 = shared-variable "My Computer\\SpoofNPSVariables.lvlib\\WT-35_S"(w239) -> ()  [unwired: 1 in, 1 out]
              n219 = shared-variable "My Computer\\SpoofNPSVariables.lvlib\\WT-40_S"(w240) -> ()  [unwired: 1 in, 1 out]
              n220 = shared-variable "My Computer\\SpoofNPSVariables.lvlib\\BT-41_S"(w241) -> ()  [unwired: 1 in, 1 out]
              n221 = shared-variable "My Computer\\SpoofNPSVariables.lvlib\\WT-42_S"(w242) -> ()  [unwired: 1 in, 1 out]
              n222 = shared-variable "My Computer\\SpoofNPSVariables.lvlib\\BT-43_S"(w243) -> ()  [unwired: 1 in, 1 out]
              n223 = Unbundle By Name(w195) -> ("[33]"=w244:sgl, "[34]"=w245:sgl, "[35]"=w246:sgl, "[36]"=w247:sgl, "[37]"=w248:sgl, "[38]"=w249:sgl, "[39]"=w250:sgl, "[40]"=w251:sgl)
              n224 = shared-variable "My Computer\\SpoofNPSVariables.lvlib\\BT-60_S"(w244) -> ()  [unwired: 1 in, 1 out]
              n225 = shared-variable "My Computer\\SpoofNPSVariables.lvlib\\WT-61_S"(w245) -> ()  [unwired: 1 in, 1 out]
              n226 = shared-variable "My Computer\\SpoofNPSVariables.lvlib\\WT-62_S"(w246) -> ()  [unwired: 1 in, 1 out]
              n227 = shared-variable "My Computer\\SpoofNPSVariables.lvlib\\BT-63_S"(w247) -> ()  [unwired: 1 in, 1 out]
              n228 = shared-variable "My Computer\\SpoofNPSVariables.lvlib\\WT-64_S"(w248) -> ()  [unwired: 1 in, 1 out]
              n229 = shared-variable "My Computer\\SpoofNPSVariables.lvlib\\BT-65_S"(w249) -> ()  [unwired: 1 in, 1 out]
              n230 = shared-variable "My Computer\\SpoofNPSVariables.lvlib\\BT-66_S"(w250) -> ()  [unwired: 1 in, 1 out]
              n231 = shared-variable "My Computer\\SpoofNPSVariables.lvlib\\WT-67_S"(w251) -> ()  [unwired: 1 in, 1 out]
              n232 = Unbundle By Name(w195) -> ("[41]"=w252:sgl, "[42]"=w253:sgl, "[43]"=w254:sgl, "[44]"=w255:sgl, "[45]"=w256:sgl, "[46]"=w257:sgl, "[47]"=w258:sgl, "[48]"=w259:sgl, "[49]"=w260:sgl, "[50]"=w261:sgl)
              n233 = Unbundle By Name(w195) -> ("[51]"=w262:sgl, "[52]"=w263:sgl)
              n234 = Unbundle By Name(w195) -> ("[57]"=w201:sgl, "[58]"=w200:sgl, "[59]"=w199:sgl, "[60]"=w198:sgl, "[61]"=w197:sgl, "[62]"=w196:sgl)
              n235 = shared-variable "My Computer\\SpoofNPSVariables.lvlib\\ST-10_S"(w252) -> ()  [unwired: 1 in, 1 out]
              n236 = shared-variable "My Computer\\SpoofNPSVariables.lvlib\\ST-11_S"(w253) -> ()  [unwired: 1 in, 1 out]
              n237 = shared-variable "My Computer\\SpoofNPSVariables.lvlib\\ST-12-N_S"(w254) -> ()  [unwired: 1 in, 1 out]
              n238 = shared-variable "My Computer\\SpoofNPSVariables.lvlib\\ST-12-SE_S"(w255) -> ()  [unwired: 1 in, 1 out]
              n239 = shared-variable "My Computer\\SpoofNPSVariables.lvlib\\ST-12-SW_S"(w256) -> ()  [unwired: 1 in, 1 out]
              n240 = shared-variable "My Computer\\SpoofNPSVariables.lvlib\\ST-13_S"(w257) -> ()  [unwired: 1 in, 1 out]
              n241 = shared-variable "My Computer\\SpoofNPSVariables.lvlib\\ST-14-N_S"(w258) -> ()  [unwired: 1 in, 1 out]
              n242 = shared-variable "My Computer\\SpoofNPSVariables.lvlib\\ST-14-E_S"(w259) -> ()  [unwired: 1 in, 1 out]
              n243 = shared-variable "My Computer\\SpoofNPSVariables.lvlib\\ST-14-S_S"(w260) -> ()  [unwired: 1 in, 1 out]
              n244 = shared-variable "My Computer\\SpoofNPSVariables.lvlib\\ST-14-W_S"(w261) -> ()  [unwired: 1 in, 1 out]
              n245 = shared-variable "My Computer\\SpoofNPSVariables.lvlib\\AT-01_S"(w262) -> ()  [unwired: 1 in, 1 out]
              n246 = shared-variable "My Computer\\SpoofNPSVariables.lvlib\\AT-02_S"(w263) -> ()  [unwired: 1 in, 1 out]
              n247 = shared-variable "My Computer\\SpoofCore_Variables.lvlib\\Desired Power_S"(w201) -> ()  [unwired: 1 in, 1 out]
              n248 = shared-variable "My Computer\\SpoofCore_Variables.lvlib\\Power Input Signal_S"(w200) -> ()  [unwired: 1 in, 1 out]
              n249 = shared-variable "My Computer\\SpoofCore_Variables.lvlib\\Power Output_S"(w199) -> ()  [unwired: 1 in, 1 out]
              n250 = shared-variable "My Computer\\SpoofVFD_Variables.lvlib\\CTAH Frequency_S"(w198) -> ()  [unwired: 1 in, 1 out]
              n251 = shared-variable "My Computer\\SpoofVFD_Variables.lvlib\\TCHX Frequency_S"(w197) -> ()  [unwired: 1 in, 1 out]
              n252 = shared-variable "My Computer\\SpoofVFD_Variables.lvlib\\Pump Frequency_S"(w196) -> ()  [unwired: 1 in, 1 out]
              n253 = Unbundle By Name(w195) -> ("[53]"=w264:sgl, "[54]"=w265:sgl, "[55]"=w266:sgl, "[56]"=w267:sgl)
              n254 = shared-variable "My Computer\\SpoofNPSVariables.lvlib\\FM-20_S"(w264) -> ()  [unwired: 1 in, 1 out]
              n255 = shared-variable "My Computer\\SpoofNPSVariables.lvlib\\FM-30_S"(w265) -> ()  [unwired: 1 in, 1 out]
              n256 = shared-variable "My Computer\\SpoofNPSVariables.lvlib\\FM-40_S"(w266) -> ()  [unwired: 1 in, 1 out]
              n257 = shared-variable "My Computer\\SpoofNPSVariables.lvlib\\FM-60_S"(w267) -> ()  [unwired: 1 in, 1 out]
            }
            frame "ns=2;s=Boolean Control Actions" {
              n258 = Variant To Data(type=bool[] [], Variant=w271) -> (data=w278:bool[])  [unwired: 1 in, 1 out]
              n259 = Array To Cluster(array=w278) -> (cluster=w277:T10)
              n260 = Unbundle By Name(w277) -> ("[0]"=w276:bool, "[1]"=w275:bool, "[2]"=w274:bool, "[3]"=w273:bool, "[4]"=w272:bool)
              n261 = shared-variable "My Computer\\RemoteVIVariables.lvlib\\Spoof Enabled"(w276) -> ()  [unwired: 1 in, 1 out]
              n262 = shared-variable "My Computer\\Core_Variables.lvlib\\Power Output On"(w275) -> ()  [unwired: 1 in, 1 out]
              n263 = shared-variable "My Computer\\VFD_Variables.lvlib\\Activate CTAH"(w274) -> ()  [unwired: 1 in, 1 out]
              n264 = shared-variable "My Computer\\VFD_Variables.lvlib\\Activate TCHX"(w273) -> ()  [unwired: 1 in, 1 out]
              n265 = shared-variable "My Computer\\VFD_Variables.lvlib\\Activate Pump"(w272) -> ()  [unwired: 1 in, 1 out]
            }
            frame "ns=2;s=Spoofed Boolean Controls" {
              n266 = Variant To Data(type=bool[] [], Variant=w280) -> (data=w287:bool[])  [unwired: 1 in, 1 out]
              n267 = Array To Cluster(array=w287) -> (cluster=w286:T10)
              n268 = Unbundle By Name(w286) -> ("[0]"=w285:bool, "[1]"=w284:bool, "[2]"=w283:bool, "[3]"=w282:bool, "[4]"=w281:bool)
              n269 = shared-variable "My Computer\\RemoteVIVariables.lvlib\\Spoof Enabled"(w285) -> ()  [unwired: 1 in, 1 out]
              n270 = shared-variable "My Computer\\SpoofCore_Variables.lvlib\\Power Output On_S"(w284) -> ()  [unwired: 1 in, 1 out]
              n271 = shared-variable "My Computer\\SpoofVFD_Variables.lvlib\\Activate CTAH_S"(w283) -> ()  [unwired: 1 in, 1 out]
              n272 = shared-variable "My Computer\\SpoofVFD_Variables.lvlib\\Activate CTAH_S"(w282) -> ()  [unwired: 1 in, 1 out]
              n273 = shared-variable "My Computer\\SpoofVFD_Variables.lvlib\\Activate Pump_S"(w281) -> ()  [unwired: 1 in, 1 out]
            }
            frame "ns=2;s=Result Boolean Controls" {
              n274 = Variant To Data(type=bool[] [], Variant=w289) -> (data=w296:bool[])  [unwired: 1 in, 1 out]
              n275 = Array To Cluster(array=w296) -> (cluster=w295:T10)
              n276 = Unbundle By Name(w295) -> ("[0]"=w294:bool, "[1]"=w293:bool, "[2]"=w292:bool, "[3]"=w291:bool, "[4]"=w290:bool)
              n277 = shared-variable "My Computer\\RemoteVIVariables.lvlib\\Spoof Enabled"(w294) -> ()  [unwired: 1 in, 1 out]
              n278 = shared-variable "My Computer\\ResultCore_Variables.lvlib\\Power Output On_R"(w293) -> ()  [unwired: 1 in, 1 out]
              n279 = shared-variable "My Computer\\ResultVFD_Variables.lvlib\\Activate CTAH_R"(w292) -> ()  [unwired: 1 in, 1 out]
              n280 = shared-variable "My Computer\\ResultVFD_Variables.lvlib\\Activate TCHX_R"(w291) -> ()  [unwired: 1 in, 1 out]
              n281 = shared-variable "My Computer\\ResultVFD_Variables.lvlib\\Activate Pump_R"(w290) -> ()  [unwired: 1 in, 1 out]
            }
          }
        }
      }
    }
    n282 = Wait (ms)(milliseconds to wait=u32 100) -> ()  [unwired: 1 out]
    n283 = Unbundle By Name(w24) -> ("status"=w29:bool)
    n284 = Not(x=w29) -> (.not. x?=w30:bool)
    n285 = shared-variable "My Computer\\RemoteVIVariables.lvlib\\Read Connection"(w30) -> ()  [unwired: 1 in, 1 out]
    n286 = shared-variable "My Computer\\RemoteVIVariables.lvlib\\Stop Reading"() -> (w27:bool)  [unwired: 1 in, 1 out]
    n287 = Build Array(w29, "stop", w27) -> (w26:bool[])
    n288 = Or Array Elements(Boolean array=w26) -> (logical OR=w25:bool)
  }
  n289 = shared-variable "My Computer\\RemoteVIVariables.lvlib\\Stop Reading"(w4) -> ()  [unwired: 1 in, 1 out]
  n290 = call <vilib>:"Delete Monitored Nodes.vi"("error in (no error)"=w1, "node IDs"=w7, "subscription ID in"=w11, "OPC UA client refnum in"=w6) -> ("error out"=w12:errorcluster, "OPC UA client refnum out"=w13:T4)  [unwired: 3 in, 3 out]
  n291 = Build Array(w11) -> (w10:T5[])
  n292 = call <vilib>:"Delete Subscriptions.vi"("error in (no error)"=w12, "subscription IDs"=w10, "OPC UA client refnum in"=w13) -> ("error out"=w14:errorcluster, "OPC UA client refnum out"=w15:T4)  [unwired: 6 in, 1 out]
  n293 = call <vilib>:"Disconnect.vi"("error in (no error)"=w14, "OPC UA client refnum in"=w15) -> ("error out"=→"error out":errorcluster)  [unwired: 9 in]
